vi "DaqAssistants2.vi"(11 "output":dbl) -> (3 "Numeric":dbl)   [LabVIEW 2017]
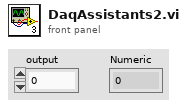
[diagram p1: front panel]
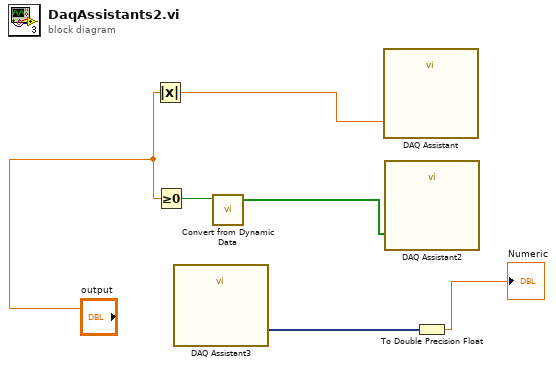
[diagram p0: block diagram]
diagram:
  n1 = Absolute Value(x="output") -> (abs(x)=w4:dbl)
  n2 = Greater Or Equal To 0?(x="output") -> (x >= 0?=w1:bool)
  n3 = call "DAQ Assistant3"() -> ("data"=w6:dynamicdata)  [unwired: 16 in, 3 out]
  n4 = call "Convert from Dynamic Data"("Dynamic Data Type"=w1) -> ("Array"=w5:bool[])  [unwired: 3 in]
  n5 = call "DAQ Assistant"("data"=w4) -> ()  [unwired: 17 in, 2 out]
  n6 = call "DAQ Assistant2"("data"=w5) -> ()  [unwired: 17 in, 2 out]
  n7 = To Double Precision Float(number=w6) -> (double precision float=→"Numeric":dbl)
